vi "Versions.vi"(8 "error in (no error)":errorcluster, 11 "Instrument Handle In":i32) -> (0 "error out":errorcluster, 1 "Driver Rev":string caption="driverRevision", 2 "ID":string, 3 "Instrument Handle Out":i32, 4 "configuration":i32[](array[numeric]))   [LabVIEW 8.6, in "ZTScopeM.lvlib"]
doc: "Query all instrument version information."
uses:
  ZTScopeM.lvlib
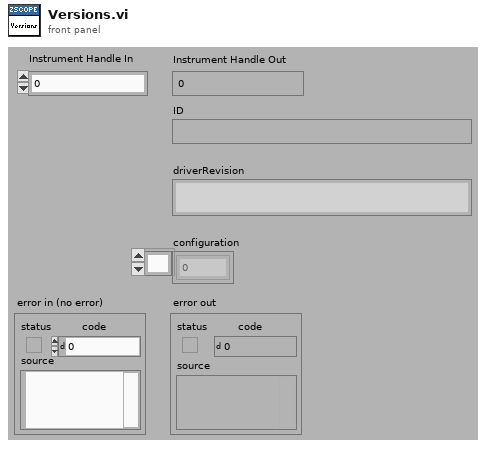
[diagram p1: front panel]
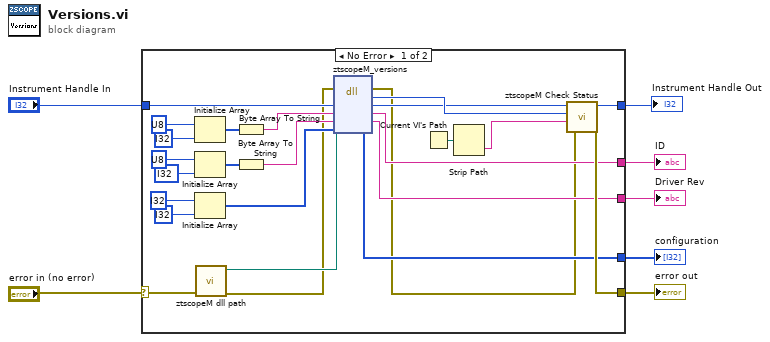
[diagram p0: block diagram]
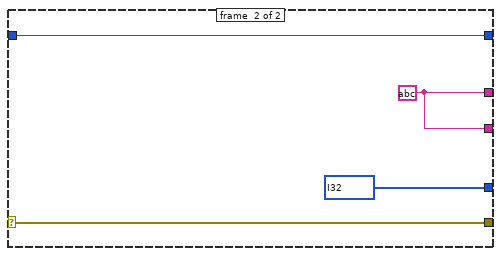
[diagram p2: hidden frame]
diagram:
  n1 = case shown="No Error" "error in (no error)" {
    selector: "error in (no error)" -> [w21 w36]
    tunnel: [w29 w36] -> w6
    tunnel: "Instrument Handle In" -> [w31 w35]
    tunnel: [w30 w35] -> w4
    tunnel: [w19 w34] -> w3
    tunnel: [w18 w34] -> w2
    tunnel: [w17 i32[] ? ("configuration")] -> w1
    frame #0 {
      n2 = Initialize Array(u8 ? ("element"), i32 ? ("dimension size")) -> (w23:u8[])
      n3 = Initialize Array(u8 ? ("element"), i32 ? ("dimension size")) -> (w16:u8[])
      n4 = Initialize Array(i32 ? ("element"), i32 ? ("dimension size")) -> (w10:i32[])
      n5 = call "ztscopeM dll path.vi"("error in (no error)"=w21) -> ("error out"=w9:errorcluster, "<instrument>.dll path"=w20:path)  [unwired: 9 in]
      n6 = Byte Array To String(unsigned byte array=w23) -> (string=w22:string)
      n7 = Byte Array To String(unsigned byte array=w16) -> (string=w13:string)
      n8 = dll-call lib="C:/Projects/codedepot/Teradyne/2016-1034 Teradyne ZScope API/Software/C src/ztScopeM/ZtScopeM.dll" fn="ztscopeM_versions"(path in=w20, error in=w9, "Instrument Handle"=w31, "ID"=w22, "driverRevision"=w13, "configuration"=w10) -> (error out=w8:errorcluster, "Status"=w27:i32, "Instrument Handle"=w26:i32, "ID"=w19:string, "driverRevision"=w18:string, "configuration"=w17:i32[])  [unwired: 1 in, 1 out]
      n9 = Current VI's Path() -> (path=w32:path)
      n10 = Strip Path(path=w32) -> (name=w28:string)  [unwired: 1 out]
      n11 = call "ztscopeM Check Status.vi"("error in"=w8, "name of VI"=w28, "status (return code)"=w27, "instrument handle in"=w26) -> ("error out"=w29:errorcluster, "instrument handle out"=w30:i32)  [unwired: 2 in]
    }
    frame #1 {
      w34 = string ?
    }
  }
  "error out" <- w6
  "Instrument Handle Out" <- w4
  "ID" <- w3
  "Driver Rev" <- w2
  "configuration" <- w1
